vi "3-1 random controllo se compreso control STOP.vi"(0 "high limit":dbl format="%.2f", 1 "low limit":dbl format="%.2f", 2 "Control (default OFF)":bool, 3 "stop":bool, 4 "Data in":dbl) -> (5 "data out":dbl format="%.2f")   [LabVIEW 2012]
doc: "© Copyright M. Ferrari 1999"
panel:
  # "Se control = ON, bisogna verificare che il valore sia compreso nei limiti\n                     trasferendo il valore di ingresso diviso per il range ( high limit-low limit)\n                     in uscita; se il valore  \"data in\"  non rientra nei limiti, oppure\nse control = OFF, non viene effettuato nessun controllo e il valore di ingresso passa\n                    direttamente in uscita"
  # "Completare il VI facendo in modo che venga eseguito ciclicamente ogni 2 sec. e che \nl' esecuzione venga terminata nel caso in cui il dato in ingresso (data in) sia > del doppio\ndi hight limit, oppure nel caso in cui venga premuto un apposito pulsante \"STOP\" (che \nandrˆ inserito nel pannello di controllo). Inoltre il dato di ingresso ( indicato con data in) \ndovrˆ essere generato automaticamente e risultare un valore casuale compreso fra 1 e 11"
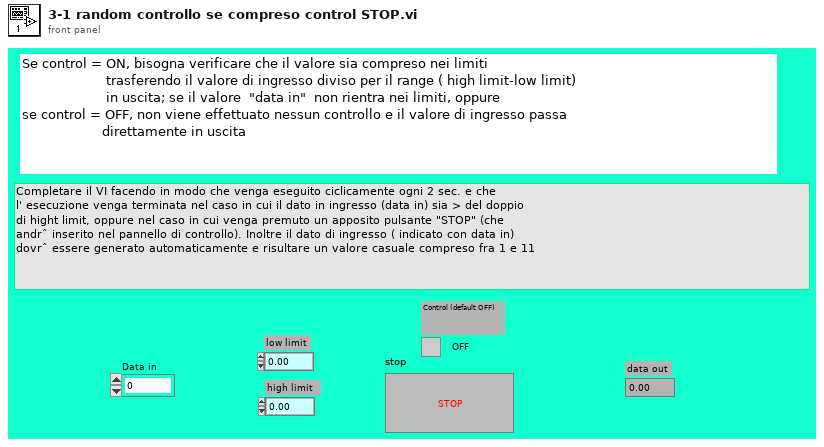
[diagram p1: front panel]
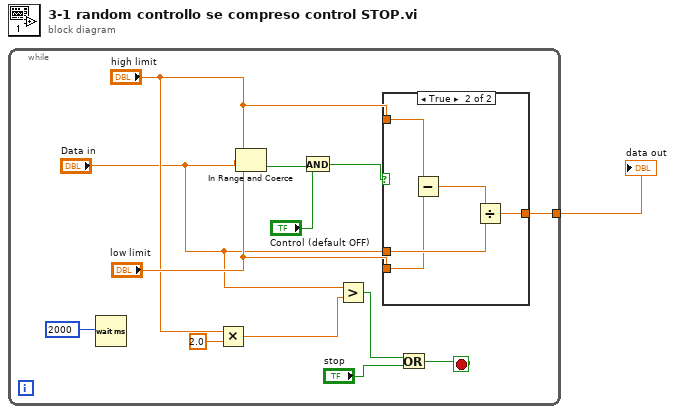
[diagram p0: block diagram]
diagram:
  n1 = while {
    tunnel: [w14] -> w1
    stop <- w10 stop-if-true
    n2 = Wait (ms)(milliseconds to wait=2000) -> ()  [unwired: 1 out]
    n3 = Multiply(x="high limit", y=2.0) -> (x*y=w4:dbl)
    n4 = In Range and Coerce(upper limit="high limit", x="Data in", lower limit="low limit") -> (In Range?=w8:bool)  [unwired: 1 out]
    n5 = And(x=w8, y="Control (default OFF)") -> (x .and. y?=w6:bool)
    n6 = Greater?(x="Data in", y=w4) -> (0:w12:bool)
    n7 = case shown="True" w6 {
      tunnel: "Data in" -> [w15 w20]
      tunnel: "high limit" -> [_ w18]
      tunnel: "low limit" -> [_ w19]
      tunnel: [w15 w16] -> w14
      frame False {
      }
      frame True {
        n8 = Subtract(x=w18, y=w19) -> (x-y=w17:dbl)
        n9 = Divide(x=w20, y=w17) -> (x/y=w16:dbl)
      }
    }
    n10 = Or(x=w12, y="stop") -> (x .or. y?=w10:bool)
  }
  "data out" <- w1
